vi "Copy.vi"(8 "error in (no error)":errorcluster, 10 "dvotTTPathPoint (to be copied)":refnum<class "dvotTTPathPoint.lvclass">, 11 "dvotTTPathPoint in":refnum<class "dvotTTPathPoint.lvclass">) -> (0 "error out":errorcluster, 2 "dvotTTPathPoint (to be copied) out":refnum<class "dvotTTPathPoint.lvclass">, 3 "dvotTTPathPoint out":refnum<class "dvotTTPathPoint.lvclass">)   [LabVIEW 2012, in "dvotTTPathPoint.lvclass"]
uses:
  dvotTTPathPoint.lvclass
  dvotTTPathPoint.lvclass/dvotTTPathPoint.ctl
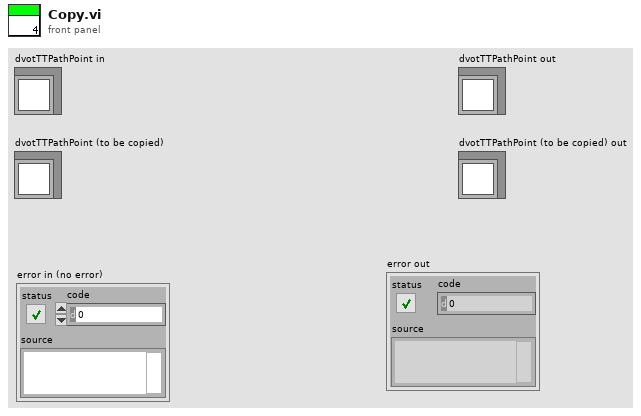
[diagram p1: front panel]
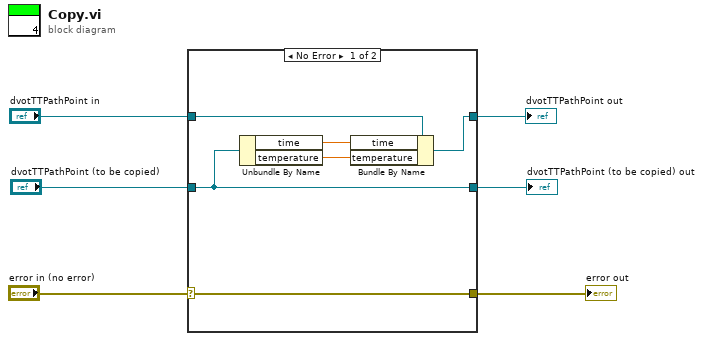
[diagram p0: block diagram]
diagram:
  n1 = case shown="No Error" "error in (no error)" {
    selector: "error in (no error)" -> [w12 w15]
    tunnel: [w12 w15] -> w5
    tunnel: "dvotTTPathPoint in" -> [w11 w14]
    tunnel: "dvotTTPathPoint (to be copied)" -> [w7 w13]
    tunnel: [w10 w14] -> w2
    tunnel: [w7 w13] -> w1
    frame No Error {
      n2 = Unbundle By Name(w7) -> ("time"=w9:dbl, "temperature"=w8:dbl)
      n3 = Bundle By Name(cluster=w11, "time"=w9, "temperature"=w8) -> (w10:refnum<class "dvotTTPathPoint.lvclass">)
    }
    frame Error {
    }
  }
  "dvotTTPathPoint out" <- w2
  "dvotTTPathPoint (to be copied) out" <- w1
  "error out" <- w5
